vi "Select Error Code Dialog.vi"(0 "state in":T1=enum."load project errors", 1 "selected error ID":string) -> (2 "state out":T1=enum."load project errors")   [LabVIEW 2016]
uses:
  Controls/Error Codes List Window States.ctl
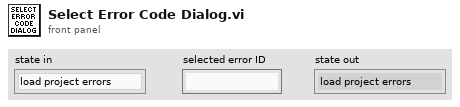
[diagram p1: front panel]
types:
  T1 = typedef "Error Codes List Window States.ctl" = enum16{"init", "load project errors", "parse combo box", "update list view", "open FP", "close", "idle", "add error", "remove error", "edit error", "edit file", "change scope", "filter"}
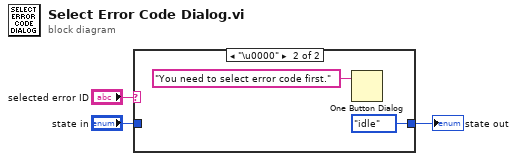
[diagram p0: block diagram]
diagram:
  n1 = case shown="\"\"" "selected error ID" {
    tunnel: [w4 Error_Codes_List_Window_States."idle" ("state in")] -> w2
    tunnel: "state in" -> [w4 _]
    frame Default {
    }
    frame "\u0000" {
      n2 = One Button Dialog(message="You need to select error code first.") -> ()  [unwired: 1 in, 1 out]
    }
  }
  "state out" <- w2
